vi "PointToRoi.vi"(8 "error in (no error)":errorcluster, 9 "ROISize":cluster{"Width":dbl, "Height":dbl}, 10 "r":dbl, 11 "Point":T1 {"Y" format="%.2f"; "X" format="%.2f"}) -> (0 "error out":errorcluster, 3 "ROI Descriptor":T2 {"Contours"."Type" items=["No Selection", "Point", "Line", "Rectangle", "Oval", "Polygon", "Freehand Region", "Annulus", "Unused2", "Unused3", "Broken Line", "Freehand Line", "Rotated Rectangle"]})   [LabVIEW 2015]
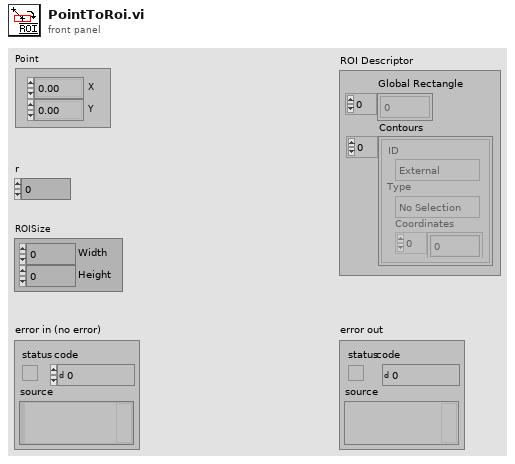
[diagram p1: front panel]
types:
  T1 = typedef "IMAQ Point" = cluster{"X":sgl, "Y":sgl}
  T2 = typedef "ROI Descriptor" = cluster{"Global Rectangle":i32[], "Contours":cluster{"ID":enum32{"External", "Internal"}, "Type":u32, "Coordinates":i32[]}[]}
  T3 = cluster{"ID":enum32{"External", "Internal"}, "Type":u32, i32[]}
  T4 = cluster{"ID":enum32{"External", "Internal"}, "Type":u32, i32[]}[]
  T5 = cluster{i32[], cluster{"ID":enum32{"External", "Internal"}, "Type":u32, i32[]}[]}
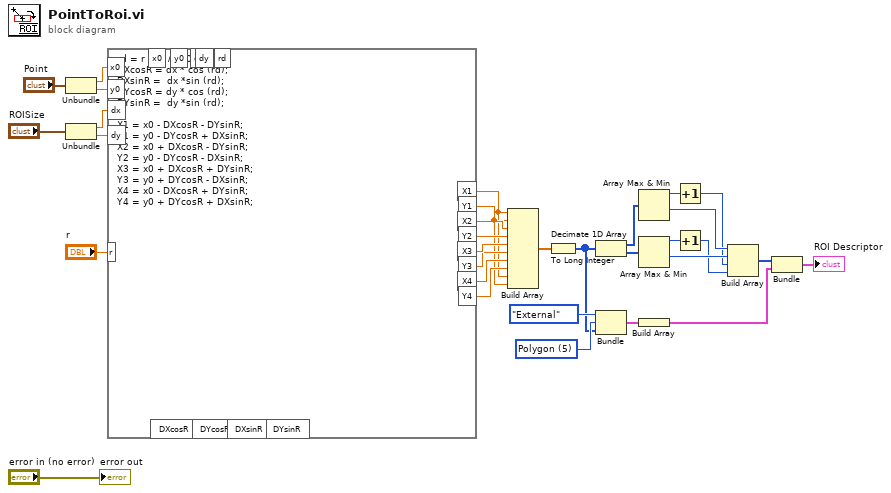
[diagram p0: block diagram]
diagram:
  w29 = u32 5 items=["No Selection", "Point", "Line", "Rectangle", "Oval", "Polygon", "Free", "Annulus", "Unused2", "Unused3", "Broken Line", "Free Hand Line", "Rotated Rectangle"] ("Type")
  n1 = Unbundle("Point") -> ("X"=w6:sgl, "Y"=w5:sgl)
  n2 = Unbundle("ROISize") -> ("Width"=w3:dbl, "Height"=w2:dbl)
  n3 = formula code="rd = r * pi / 180.0;\nDXcosR = dx * cos (rd);\nDXsinR =  dx *sin (rd);\nDYcosR = dy * cos (rd);\nDYsinR =  dy *sin (rd);\n\nX1 = x0 - DXcosR - DYsinR;\nY1 = y0 - DYcosR + DXsinR;\nX2 = x0 + DXcosR - DYsinR;\nY2 = y0 - DYcosR - DXsinR;\nX3 = x0 + DXcosR + DYsinR;\nY3 = y0 + DYcosR - DXsinR;\nX4 = x0 - DXcosR + DYsinR;\nY4 = y0 + DYcosR + DXsinR;"("r"="r", "x0"=w6, "y0"=w5, "dx"=w3, "dy"=w2) -> ("X1"=w12:dbl, "Y1"=w11:dbl, "X2"=w24:dbl, "Y2"=w23:dbl, "X3"=w22:dbl, "Y3"=w21:dbl, "X4"=w20:dbl, "Y4"=w19:dbl)  [unwired: 9 out]
  n4 = Build Array(w12, w11, w24, w23, w22, w21, w20, w19, w12, w11) -> (w18:dbl[])
  n5 = To Long Integer(number=w18) -> (32bit integer=w17:i32[])
  n6 = Decimate 1D Array(w17) -> (w13:i32[], w14:i32[])
  n7 = Bundle("ID"=enum32{"External", "Internal"}."External", "Type"=w29, w17) -> (w31:T3)  [unwired: 1 out]
  n8 = Array Max & Min(array=w13) -> (max value=w26:i32, min value=w28:i32)  [unwired: 2 out]
  n9 = Array Max & Min(array=w14) -> (max value=w25:i32, min value=w27:i32)  [unwired: 2 out]
  n10 = Build Array(w31) -> (w32:T4)
  n11 = Increment(x=w26) -> (x+1=w9:i32)
  n12 = Increment(x=w25) -> (x+1=w8:i32)
  n13 = Build Array(w28, w27, w9, w8) -> (w16:i32[])
  n14 = Bundle(w16, w32) -> (→"ROI Descriptor":T5)  [unwired: 1 out]
  "error out" <- "error in (no error)"
